vi "Generate RPC Methods.vi"(7 "RPC Method Parameters":T1[](array[typedef]), 8 "error in (no error)":errorcluster, 11 "Server class in":refnum<vi>) -> (0 "error out":errorcluster, 3 "Server class out":refnum<vi>)   [LabVIEW 2019, in "gRPC Scripting Tools.lvlib"]
uses:
  gRPC Scripting Tools.lvlib
  TypeDefs/RPC Method Parameters.ctl
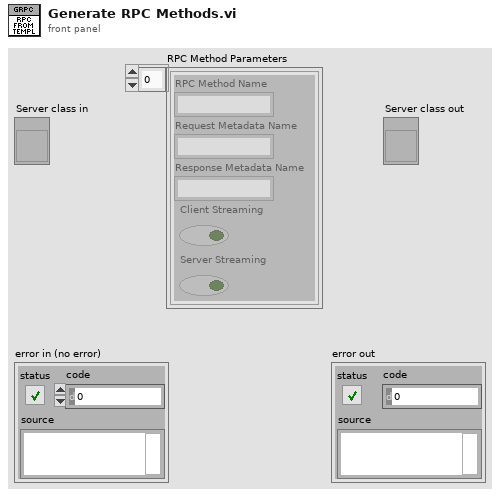
[diagram p1: front panel]
types:
  T1 = typedef "gRPC Scripting Tools.lvlib/RPC Method Parameters.ctl" = cluster{"RPC Method Name":string, "Request Metadata Name":string, "Response Metadata Name":string, "Client Streaming":bool, "Server Streaming":bool}
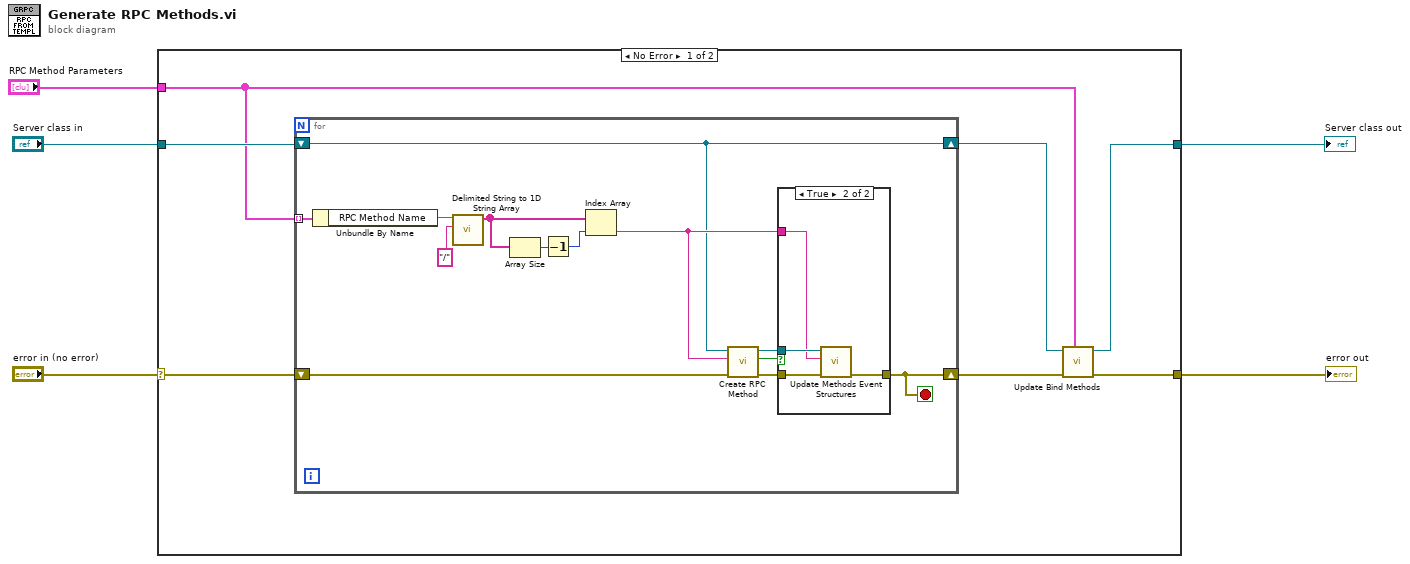
[diagram p0: block diagram]
diagram:
  n1 = case shown="No Error" "error in (no error)" {
    selector: "error in (no error)" -> [w12 w32]
    tunnel: [w8 w32] -> w5
    tunnel: "Server class in" -> [w11 w31]
    tunnel: [w6 w31] -> w2
    tunnel: "RPC Method Parameters" -> [w9 _]
    frame No Error {
      n2 = for {
        tunnel: w9 -> [w19] mode=indexing
        shift-right: [w14] -> w10
        shift-left: w12 -> [w25]
        shift-right: [w13] -> w7
        shift-left: w11 -> [w13]
        stop <- w14 stop-if-true
        n3 = Unbundle By Name(w19) -> ("RPC Method Name"=w21:string)
        n4 = call <vilib>:"Delimited String to 1D String Array.vi"("delimiter"="/", "delimited string"=w21) -> ("string array"=w24:string[])  [unwired: 9 in]
        n5 = Array Size(array=w24) -> (size(s)=w22:i32)
        n6 = Decrement(x=w22) -> (x-1=w23:i32)
        n7 = Index Array(array=w24, index=w23) -> (element=w15:string)
        n8 = call "Create RPC Method.vi"("error in (no error)"=w25, "RPC Method Name"=w15, "Server class in"=w13) -> ("error out"=w18:errorcluster, "Newly created ?"=w16:bool, "Server class out"=w17:refnum<vi>)  [unwired: 6 in]
        n9 = case shown="True" w16 {
          tunnel: w18 -> [w26 w30]
          tunnel: w17 -> [_ w29]
          tunnel: w15 -> [_ w28]
          tunnel: [w26 w27] -> w14
          frame False {
          }
          frame True {
            n10 = call "Update Methods Event Structures.vi"("error in (no error)"=w30, "RPC Method Name"=w28, "LVClassLibrary in"=w29) -> ("error out"=w27:errorcluster)  [unwired: 7 in, 1 out]
          }
        }
      }
      n11 = call "Update Bind Methods.vi"("RPC Method Parameters"=w9, "error in (no error)"=w10, "Server class in"=w7) -> ("error out"=w8:errorcluster, "Server class out"=w6:refnum<vi>)  [unwired: 7 in]
    }
    frame Error {
    }
  }
  "error out" <- w5
  "Server class out" <- w2
